vi "Configure Report Type.vi"(0 "VISA resource name":refnum<visa-resource-name>, 1 "Hour (0)":i32 min=0 max=23 step=1, 2 "Minute (0)":i32 min=0 max=59 step=1, 5 "Report Type (0: Off)":i32(ring) items=["Off", "Hourly + Daily", "Daily + Weekly", "Daily + Monthly", "Batch", "Daily Custom"], 7 "Day (1)":i32=1 min=1 max=28 step=1, 9 "Day of Week (0: Sunday)":i32(ring) items=["Sunday", "Monday", "Tuesday", "Wednesday", "Thursday", "Friday", "Saturday"], 11 "error in (no error)":errorcluster, 12 "Save Interval (4: 10min)":i32(ring)=4 items=["2min", "3min", "4min", "5min", "10min", "15min", "30min", "1h"], 13 "File Creation Interval (0: 4h)":i32(ring) items=["4h", "6h", "8h", "12h", "24h"]) -> (4 "VISA resource name out":refnum<visa-resource-name>, 15 "error out":errorcluster)   [LabVIEW 2020, in "Yokogawa GX Series.lvlib"]
doc: "Sets the type of data to record.\n\nCommand: SMemory"
uses:
  <instrlib>/Yokogawa GX Series/Yokogawa GX Series.lvlib
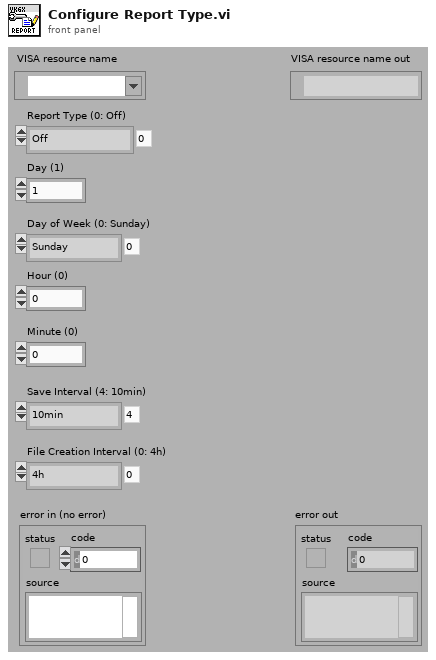
[diagram p1: front panel]
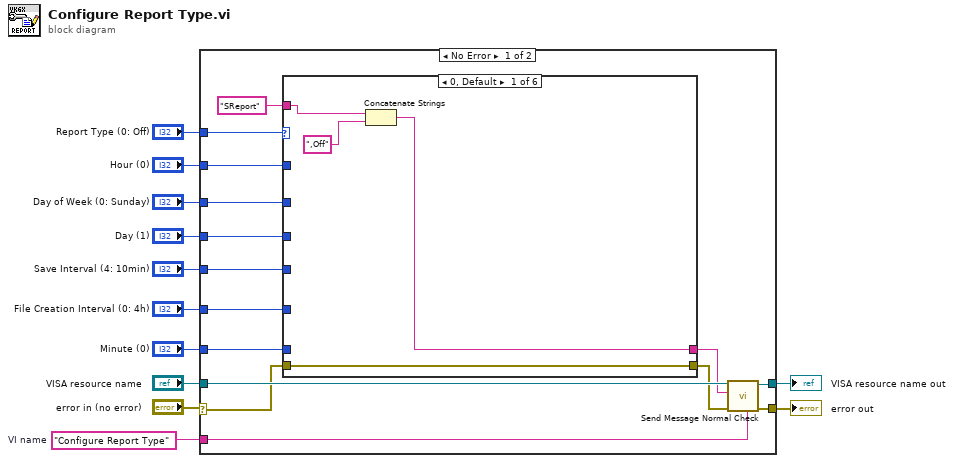
[diagram p0: block diagram]
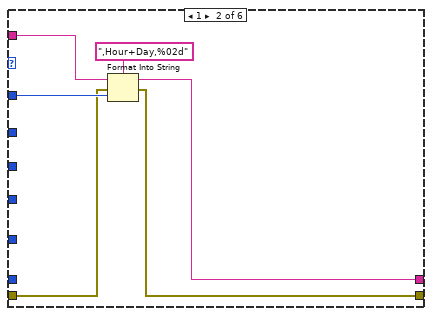
[diagram p2: hidden frame]
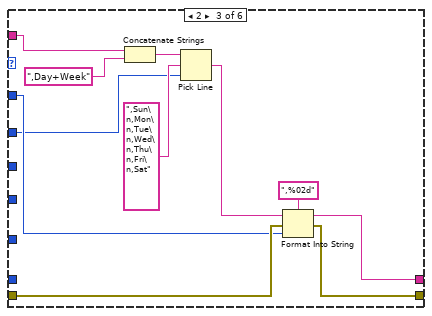
[diagram p3: hidden frame]
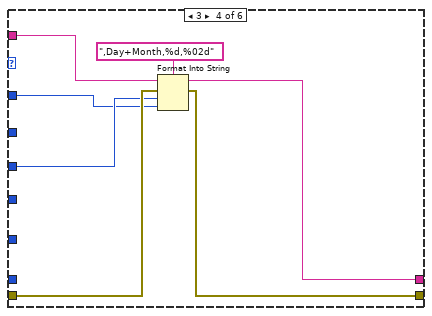
[diagram p4: hidden frame]
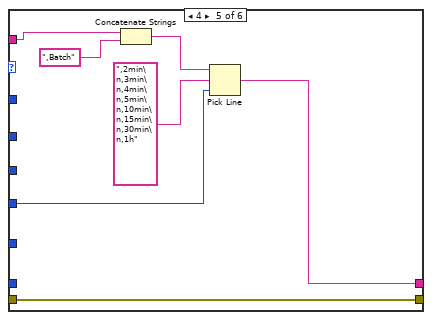
[diagram p5: hidden frame]
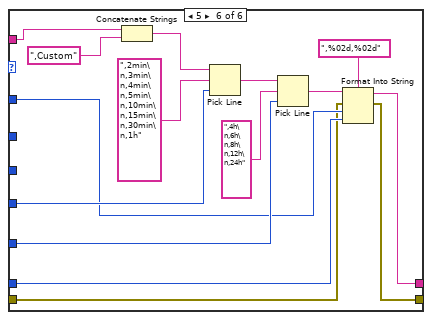
[diagram p6: hidden frame]
diagram:
  w11 = "Configure Report Type"  # VI name
  n1 = case shown="No Error" "error in (no error)" {
    selector: "error in (no error)" -> [w15 w78]
    tunnel: "VISA resource name" -> [w27 w79]
    tunnel: w11 -> [w24 _]
    tunnel: [w26 w79] -> w10
    tunnel: [w25 w78] -> w9
    tunnel: "Report Type (0: Off)" -> [w23 _]
    tunnel: "Hour (0)" -> [w21 _]
    tunnel: "Day of Week (0: Sunday)" -> [w20 _]
    tunnel: "Day (1)" -> [w19 _]
    tunnel: "Save Interval (4: 10min)" -> [w18 _]
    tunnel: "File Creation Interval (0: 4h)" -> [w17 _]
    tunnel: "Minute (0)" -> [w16 _]
    frame No Error {
      n2 = case shown="0, Default" w23 {
        tunnel: "SReport" -> [w31 w37 w43 w55 w61 w77]
        tunnel: w21 -> [_ w35 w44 w49 _ w67]
        tunnel: w20 -> [_ _ w39 _ _ _]
        tunnel: w19 -> [_ _ _ w50 _ _]
        tunnel: w18 -> [_ _ _ _ w58 w74]
        tunnel: w17 -> [_ _ _ _ _ w70]
        tunnel: w16 -> [_ _ _ _ _ w66]
        tunnel: w15 -> [w29 w34 w47 w53 w62 w65]
        tunnel: [w29 w33 w46 w52 w62 w64] -> w14
        tunnel: [w28 w32 w45 w51 w56 w63] -> w13
        frame 0, Default {
          n3 = Concatenate Strings(w31, ",Off") -> (w28:string)
        }
        frame 1 {
          n4 = Format Into String(format string=",Hour+Day,%02d", initial string=w37, error in=w34, w35) -> (resulting string=w32:string, error out=w33:errorcluster)
        }
        frame 2 {
          n5 = Concatenate Strings(w43, ",Day+Week") -> (w41:string)
          n6 = Pick Line(string ("")=w41, multi-line string=",Sun\n,Mon\n,Tue\n,Wed\n,Thu\n,Fri\n,Sat", line index=w39) -> (output string=w38:string)
          n7 = Format Into String(format string=",%02d", initial string=w38, error in=w47, w44) -> (resulting string=w45:string, error out=w46:errorcluster)
        }
        frame 3 {
          n8 = Format Into String(format string=",Day+Month,%d,%02d", initial string=w55, error in=w53, w50, w49) -> (resulting string=w51:string, error out=w52:errorcluster)
        }
        frame 4 {
          n9 = Concatenate Strings(w61, ",Batch") -> (w59:string)
          n10 = Pick Line(string ("")=w59, multi-line string=",2min\n,3min\n,4min\n,5min\n,10min\n,15min\n,30min\n,1h", line index=w58) -> (output string=w56:string)
        }
        frame 5 {
          n11 = Concatenate Strings(w77, ",Custom") -> (w75:string)
          n12 = Pick Line(string ("")=w75, multi-line string=",2min\n,3min\n,4min\n,5min\n,10min\n,15min\n,30min\n,1h", line index=w74) -> (output string=w72:string)
          n13 = Pick Line(string ("")=w72, multi-line string=",4h\n,6h\n,8h\n,12h\n,24h", line index=w70) -> (output string=w69:string)
          n14 = Format Into String(format string=",%02d,%02d", initial string=w69, error in=w65, w67, w66) -> (resulting string=w63:string, error out=w64:errorcluster)
        }
      }
      n15 = call <instrlib>:"Send Message Normal Check.vi"("Source (\"\")"=w24, "error in (no error)"=w14, "Send Message (\"\")"=w13, "VISA resource name"=w27) -> ("error out"=w25:errorcluster, "VISA resource name out"=w26:refnum<visa-resource-name>)  [unwired: 2 in, 4 out]
    }
    frame Error {
    }
  }
  "error out" <- w9
  "VISA resource name out" <- w10
